vi "ConfigInstr.vi"(6 "InstrumentName":string, 7 "VisaRessIn":refnum<visa-resource-name>, 8 "error in (no error)":errorcluster caption="entrée d'erreur (pas d'erreur)", 9 "FirstClassInst":bool, 10 "Function":string, 11 "GenData In":refnum<class "ThorCCS200.lvclass"> caption="DNL_LabVIEW Object in") -> (0 "error out":errorcluster caption="sortie d'erreur", 3 "GenData Out":refnum<class "ThorCCS200.lvclass"> caption="DNL_LabVIEW Object out")   [LabVIEW 2019, in "ThorCCS200.lvclass"]
uses:
  ThorCCS200.lvclass
  C:/Programmes Labview/LabScanV1A/DevicesClass/BaseDevice/BaseDevice.lvclass
  ThorCCS200_Func.ctl
  ThorCCS200.lvclass/ThorCCS200.ctl
  BaseDevice/BaseDevice.lvclass/BaseDevice.ctl
  BaseDevice/Accessor/SetShowInstrNm.vi
  BaseDevice/Accessor/SetInstrParam.vi
panel:
  in  "Class_Func":T1
  out "VisaRessOut":refnum<visa-resource-name>
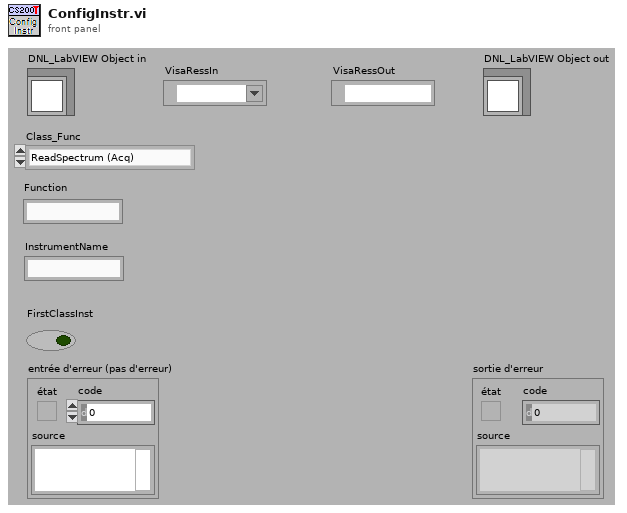
[diagram p1: front panel]
types:
  T1 = typedef "ThorCCS200.lvclass/ThorCCS200_Func.ctl" = enum16{"ReadSpectrum (Acq)"}
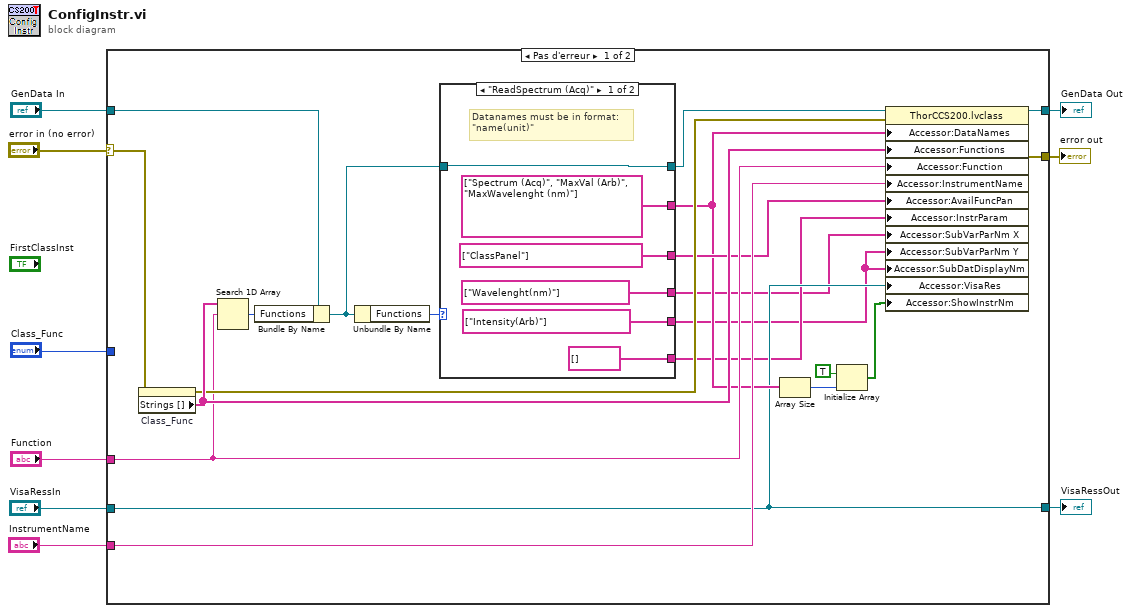
[diagram p0: block diagram]
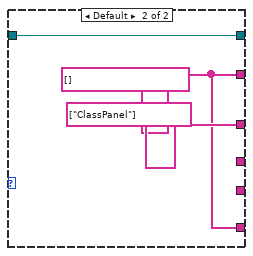
[diagram p2: hidden frame]
diagram:
  n1 = case shown="Pas d'erreur" "error in (no error)" {
    selector: "error in (no error)" -> [w24 w41]
    tunnel: [w30 w41] -> w8
    tunnel: "GenData In" -> [w25 w40]
    tunnel: [w29 w40] -> w6
    tunnel: "Class_Func" -> [_ _]
    tunnel: "Function" -> [w20 _]
    tunnel: "InstrumentName" -> [w19 _]
    tunnel: "VisaRessIn" -> [w13 _]
    tunnel: [w13 _] -> w1
    frame No Error {
      n2 = property on="Class_Func" class="Énum (strict)"(error in=w24) -> (error out=w23:errorcluster, "Strings []"=w27:string[])  [unwired: 1 in, 1 out]
      n3 = Search 1D Array(1D array=w27, element=w20) -> (index of element=w26:i32)  [unwired: 1 in]
      n4 = Bundle By Name(cluster=w25, "Functions"=w26) -> (w22:refnum<class "ThorCCS200.lvclass">)
      n5 = Unbundle By Name(w22) -> ("Functions"=w28:T1)
      n6 = case shown="\"ReadSpectrum (Acq)\"" w28 {
        tunnel: [string[] ["Spectrum (Acq)", "MaxVal (Arb)", "MaxWavelenght (nm)"] w37] -> w15
        tunnel: w22 -> [w36 w39]
        tunnel: [w36 w39] -> w21
        tunnel: [string[] ["ClassPanel"] string[] ["ClassPanel"]] -> w18
        tunnel: [string[] [] w37] -> w12
        tunnel: [string[] ["Intensity(Arb)"] _] -> w11
        tunnel: [string[] ["Wavelenght(nm)"] _] -> w10
        frame "ReadSpectrum (Acq)" {
          # "Datanames must be in format:\n\"name(unit)\""
        }
        frame Default {
          w37 = string[] []
        }
      }
      n7 = Array Size(array=w15) -> (size(s)=w17:i32)
      n8 = Initialize Array(TRUE, w17) -> (w14:bool[])
      n9 = property class="ThorCCS200.lvclass"(reference=w21, error in=w23, "Accessor:DataNames"=w15, "Accessor:Functions"=w27, "Accessor:Function"=w20, "Accessor:InstrumentName"=w19, "Accessor:AvailFuncPan"=w18, "Accessor:InstrParam"=w12, "Accessor:SubVarParNm X"=w10, "Accessor:SubVarParNm Y"=w11, "Accessor:SubDatDisplayNm"=w11, "Accessor:VisaRes"=w13, "Accessor:ShowInstrNm"=w14) -> (reference out=w29:refnum<class "ThorCCS200.lvclass">, error out=w30:errorcluster)
    }
    frame Error {
    }
  }
  "error out" <- w8
  "GenData Out" <- w6
  "VisaRessOut" <- w1
